vi "1 PulseGeneration.vi"(2 "PulseGen Packet":u64, 4 "PulseGen Ch":refnum<k21>="Connector0/DIO4") -> ()   [LabVIEW 2010]
uses:
  <vilib>/eio/EIONode/EIONode.xnode
  <vilib>/rvi/eio/nirviEIOImplementation/nirviEIOImplementation.xnode
  <vilib>/rvi/eio/common/nirviEmuClasses.ctl
  <vilib>/rvi/eio/common/nirviEmuTemplateMethod_noerrors.vi
  <vilib>/NI Veristand/FPGA/NI_VS FPGA Support.lvlib
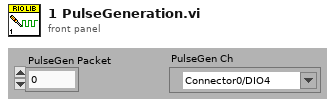
[diagram p1: front panel]
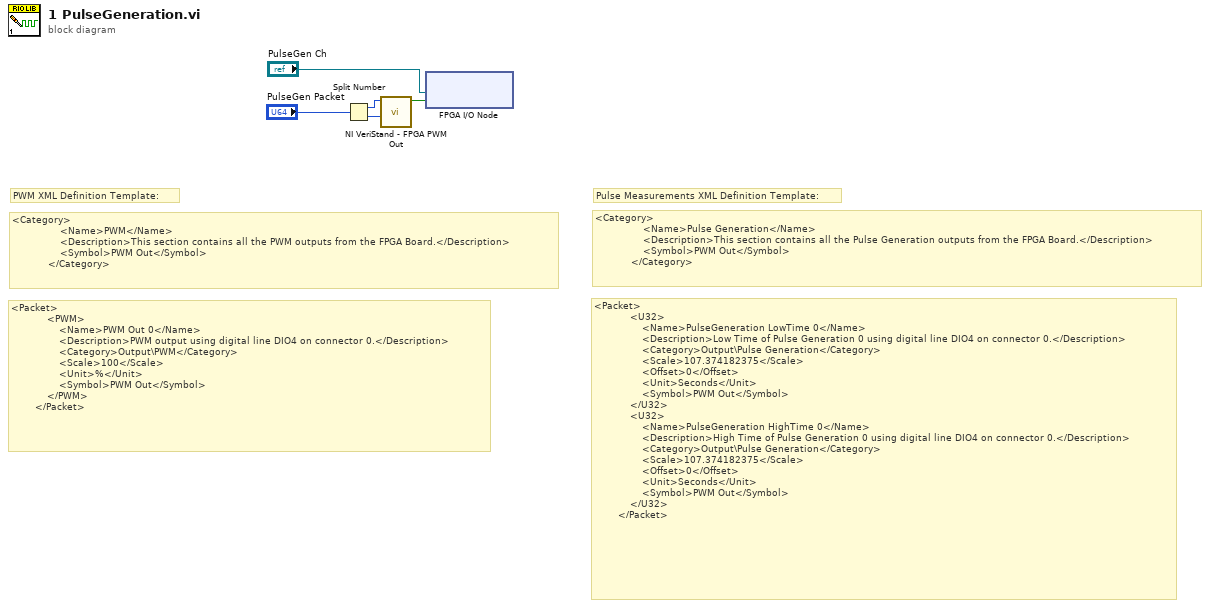
[diagram p0: block diagram]
diagram:
  # "<Category>\n                <Name>Pulse Generation</Name>\n                <Description>This section contains all the Pulse Generation outputs from the FPGA Board.</Description>\n                <Symbol>PWM Out</Symbol>\n            </Category>"
  # "<Category>\n                <Name>PWM</Name>\n                <Description>This section contains all the PWM outputs from the FPGA Board.</Description>\n                <Symbol>PWM Out</Symbol>\n            </Category>"
  # "<Packet>\n            <U32>\n                <Name>PulseGeneration LowTime 0</Name>\n                <Description>Low Time of Pulse Generation 0 using digital line DIO4 on connector 0.</Description>\n                <Category>Output\\Pulse Generation</Category>\n                <Scale>107.374182375</Scale>\n                <Offset>0</Offset>\n                <Unit>Seconds</Unit>\n                <Symbol>PWM Out</Symbol>\n            </U32>\n            <U32>\n                <Name>PulseGeneration HighTime 0</Name>\n                <Description>High Time of Pulse Generation 0 using digital line DIO4 on connector 0.</Description>\n                <Category>Output\\Pulse Generation</Category>\n                <Scale>107.374182375</Scale>\n                <Offset>0</Offset>\n                <Unit>Seconds</Unit>\n                <Symbol>PWM Out</Symbol>\n            </U32>\n        </Packet>"
  # "<Packet>\n            <PWM>\n                <Name>PWM Out 0</Name>\n                <Description>PWM output using digital line DIO4 on connector 0.</Description>\n                <Category>Output\\PWM</Category>\n                <Scale>100</Scale>\n                <Unit>%</Unit>\n                <Symbol>PWM Out</Symbol>\n            </PWM>\n        </Packet>"
  # "Pulse Measurements XML Definition Template:"
  # "PWM XML Definition Template:"
  n1 = Split Number(x="PulseGen Packet") -> (hi(x)=w4:u32, lo(x)=w5:u32)
  n2 = call <vilib>:"NI VeriStand - FPGA PWM Out.vi"("_Low Time"=w5, "_High Time"=w4) -> ("Output"=w3:bool)  [unwired: 1 in, 8 out]
  n3 = xnode "FPGA I/O Node"("I/O Item"=w3, "FPGA I/O In"="PulseGen Ch") -> ()  [unwired: 1 out]
